vi "Update Alias in Variable Table.vi"(9 "Device Name":string, 10 "Value":string, 11 "Var Name":string) -> ()   [LabVIEW 2013]
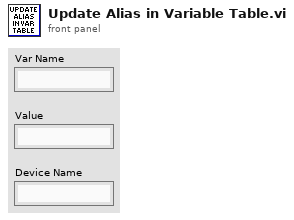
[diagram p1: front panel]
types:
  T1 = typedef "mysql_authentication.ctl" = cluster{"User":string, "Password":string, "Database":string}
  T2 = cluster{"Port":u16, "IP Address":string, "Authentication":T1}
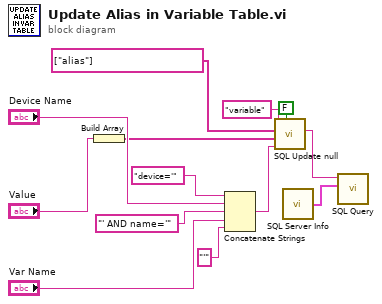
[diagram p0: block diagram]
diagram:
  n1 = Build Array("Value") -> (w5:string[])
  n2 = Concatenate Strings("device='" ("string"), "Device Name", "' AND name='" ("string"), "Var Name", "'" ("string")) -> (w12:string)
  n3 = call "SQL Update null.vi"("Use Empty String as Ignore? (T)"=FALSE, "Where clause"=w12, "Values"=w5, "Column Names"=string[] ["alias"], "Table"="variable") -> ("Query String"=w6:string)  [unwired: 6 in]
  n4 = call "SQL Server Info.vi"() -> ("SQL Server Info"=w1:T2)
  n5 = call "SQL Query.vi"("SQL Server Info"=w1, "Query"=w6) -> ()  [unwired: 8 in, 2 out]
